vi "MCP2221_SetGpioDirection.vi"(8 "error in":errorcluster, 9 "handle in":i32, 11 "direction":bool[](array[boolean])) -> (0 "error out":errorcluster, 1 "handle out":i32, 3 "return type":i32)   [LabVIEW 2025]
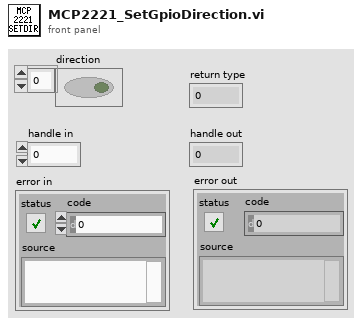
[diagram p1: front panel]
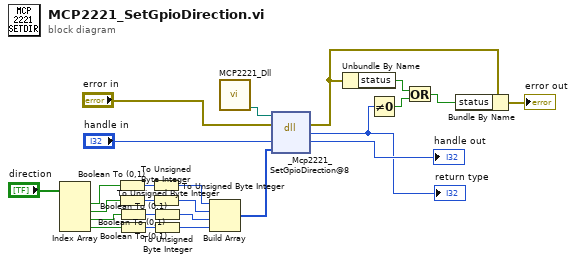
[diagram p0: block diagram]
diagram:
  n1 = Index Array(array="direction") -> (element #1=w3:bool, element #2=w4:bool, element #3=w5:bool, element #4=w6:bool)  [unwired: 4 in]
  n2 = Boolean To (0,1)(Boolean=w3) -> (0, 1=w14:i16)
  n3 = Boolean To (0,1)(Boolean=w4) -> (0, 1=w13:i16)
  n4 = Boolean To (0,1)(Boolean=w5) -> (0, 1=w12:i16)
  n5 = Boolean To (0,1)(Boolean=w6) -> (0, 1=w11:i16)
  n6 = To Unsigned Byte Integer(number=w14) -> (unsigned 8bit integer=w10:u8)
  n7 = To Unsigned Byte Integer(number=w13) -> (unsigned 8bit integer=w9:u8)
  n8 = To Unsigned Byte Integer(number=w12) -> (unsigned 8bit integer=w8:u8)
  n9 = To Unsigned Byte Integer(number=w11) -> (unsigned 8bit integer=w7:u8)
  n10 = Build Array(w10, w9, w8, w7) -> (w2:u8[])
  n11 = call "MCP2221_Dll.vi"() -> ("dll path"=w21:path)  [unwired: 11 in]
  n12 = dll-call lib="?" fn="_Mcp2221_SetGpioDirection@8"(path in=w21, error in="error in", "handle"="handle in", "direction"=w2) -> (error out=w17:errorcluster, "return type"=w15:i32, "handle"=→"handle out":i32)  [unwired: 2 in, 1 out]
  "return type" <- w15
  n13 = Unbundle By Name(w17) -> ("status"=w20:bool)
  n14 = Not Equal To 0?(x=w15) -> (x != 0?=w18:bool)
  n15 = Or(x=w20, y=w18) -> (x .or. y?=w19:bool)
  n16 = Bundle By Name(cluster=w17, "status"=w19) -> (→"error out":errorcluster)
